vi "Write-DESKTOP-V5KJPJM.vi"(8 "error in (no error)":errorcluster, 9 "Data":u8[](array[numeric]), 10 "I2C Slave Address":u8, 11 "I2C Linx in":refnum<class "LinxI2C.lvclass">) -> (0 "error out":errorcluster, 3 "I2C Linx out":refnum<class "LinxI2C.lvclass">)   [LabVIEW 2014, in "LinxI2C.lvclass"]
doc: "Write data bytes to the I2C slave device identified by I2C Slave Address."
uses:
  LinxI2C.lvclass
  LinxI2C.lvclass/LinxI2C.ctl
  <vilib>/MakerHub/LINX/Private/Local IO/LinxI2cWrite.vi
  <vilib>/MakerHub/LINX/Public/Utilities/Check Channel.vi
  <vilib>/MakerHub/LINX/Private/Local IO/Handle Errors.vi
  <vilib>/MakerHub/LINX/Private/Utilties/Generate Error.vi
  <vilib>/MakerHub/LINX/LMH-LINX.lvlib
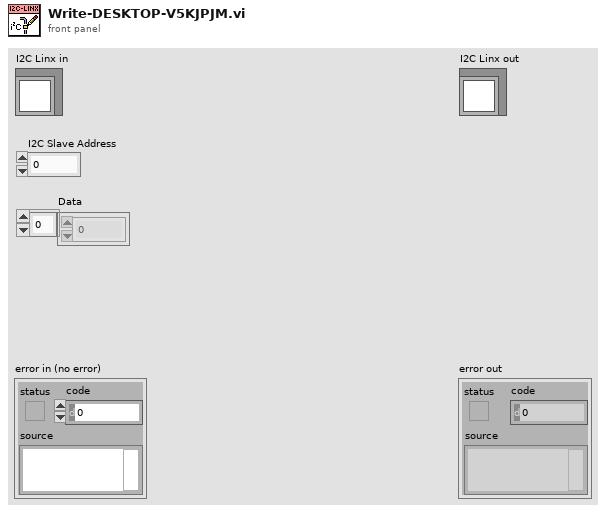
[diagram p1: front panel]
types:
  T1 = typedef "LMH-LINX.lvlib/LINX Ref.ctl" = cluster{"IO":T2, "Interface":T3, "LINX Device Config":T4}
  T2 = typedef "LMH-LINX.lvlib/Platform.ctl" = enum16{"Remote", "Local"}
  T3 = typedef "LMH-LINX.lvlib/Interface.ctl" = enum16{"Serial", "TCP"}
  T4 = typedef "LMH-LINX.lvlib/Device.lvlib/LINX Device Config.ctl" = cluster{"Interface":T3, "COM Port":refnum<visa-resource-name>, "TCP Configuration":T5, "Device Family":u8, "Device ID":u8, "Device Name":string, "TCP Ref":refnum<k5>, "Channels":T6}
  T5 = typedef "LMH-LINX.lvlib/Device.lvlib/TCP Config.ctl" = cluster{"IP Address":string, "Port":u16}
  T6 = typedef "LMH-LINX.lvlib/Channels.ctl" = cluster{"DI":u8[], "DO":u8[], "AI":u8[], "AO":u8[], "PWM":u8[], "QE":u8[], "UART":u8[], "I2C 2":u8[], "SPI":u8[], "CAN":u8[], "Servo":u8[], "AI Ref (V)":dbl, "AI Resolution (Bits)":u8, "AO Ref (V)":dbl, "AO Resolution (Bits)":u8}
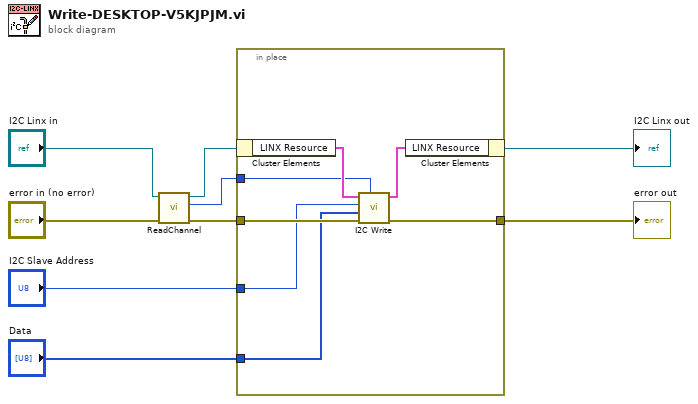
[diagram p0: block diagram]
diagram:
  n1 = call-dynamic "ReadChannel.vi"("error in (no error)"="error in (no error)", "I2C in"="I2C Linx in") -> ("error out"=w8:errorcluster, "I2C Channel"=w4:u8, "I2C out"=w6:refnum<class "LinxI2C.lvclass">)  [unwired: 7 in]
  n2 = in-place {
    in-place-border: w8 -> [w16]
    in-place-border: [w10] -> w2
    in-place-border: "I2C Slave Address" -> [w15]
    in-place-border: w4 -> [w12]
    in-place-border: "Data" -> [w11]
    n3 = in-place-cluster #1(w6) -> ("LINX Resource"=w14:T1)
    n4 = call <vilib>:"I2C Write.vi"("I2C Channel"=w12, "Error In"=w16, "Data"=w11, "I2C Slave Address (0)"=w15, "LINX Resource"=w14) -> ("Error Out"=w10:errorcluster, "LINX Resource"=w13:T1)  [unwired: 5 in]
    n5 = in-place-cluster #1("LINX Resource"=w13) -> (→"I2C Linx out":refnum<class "LinxI2C.lvclass">)
  }
  "error out" <- w2
